vi "Process.vi"(8 "error in (no error)":errorcluster, 10 "Pound in":refnum<class "Pound.lvclass">, 11 "Qbus in":refnum<class "Qbus.lvclass">) -> (0 "error out":errorcluster)   [LabVIEW 2017, in "EmsaFPGABitfileManager.lvlib"]
uses:
  <vilib>/addons/InsightCM/Devices/Shared/Emsa/EmsaFPGABifileManager/EmsaFPGABitfileManager.lvlib
  <vilib>/addons/Qbus/Qbus.lvclass
  <vilib>/NI/Software Watchdog/Pound/Pound.lvclass
  <vilib>/addons/InsightCM/Devices/Shared/Emsa/EmsaFPGABifileManager/controls/config.ctl
  <vilib>/addons/TraceLogger/TraceLogger.lvlib
  <vilib>/NI/Software Watchdog/Watchdog/Watchdog.lvclass
  <vilib>/addons/InsightCM/Devices/Shared/Common/FpgaBitfileManager/FpgaBitfileManager.lvlib
  <vilib>/rvi/interface/nirviCloseFPGA/nirviCloseFPGA.xnode
  <vilib>/FPGAPlugInAG/Dynamic/niLvFpga_Close_Dynamic.vi
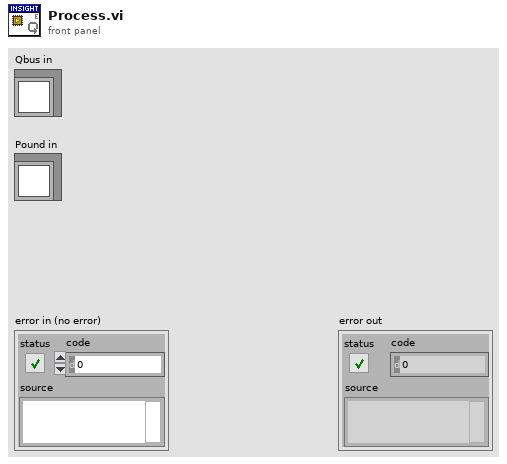
[diagram p1: front panel]
types:
  T1 = typedef "EmsaFPGABitfileManager.lvlib/config.ctl" = cluster{"FPGA VI Reference":refnum<k20>}
  T2 = typedef "cRIODetectHW.lvlib/SystemHW.ctl" = cluster{"controller":T3, "chassis":T3, "modules":T3[]}
  T3 = typedef "cRIODetectHW.lvlib/cRIO Product Info.ctl" = cluster{"vendorName":string, "productName":string, "serialNumber":string}
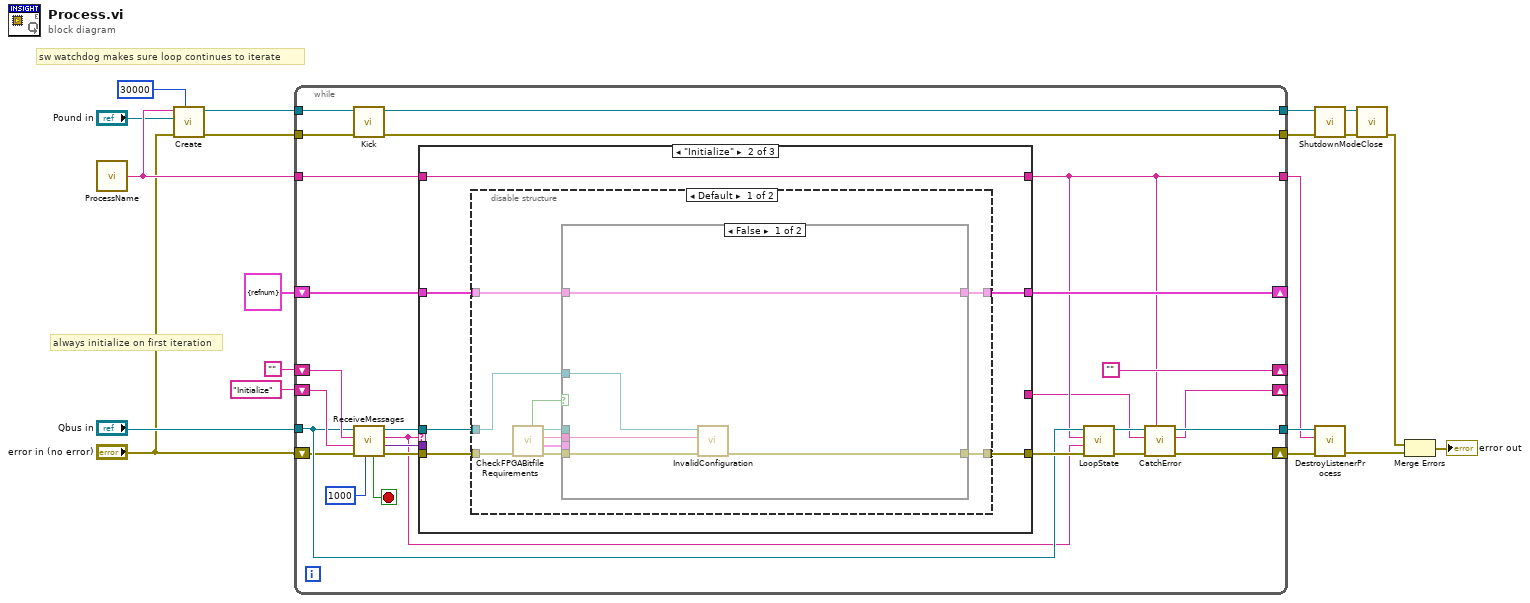
[diagram p0: block diagram]
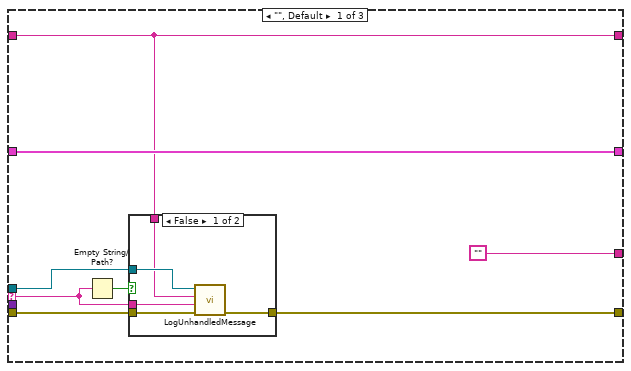
[diagram p2: hidden frame]
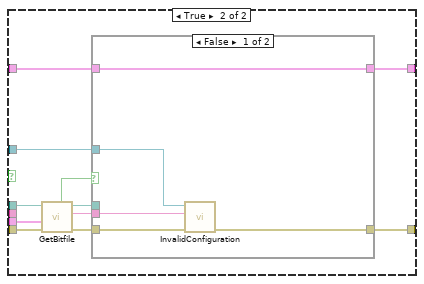
[diagram p4: hidden frame]
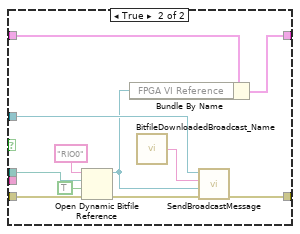
[diagram p5: hidden frame]
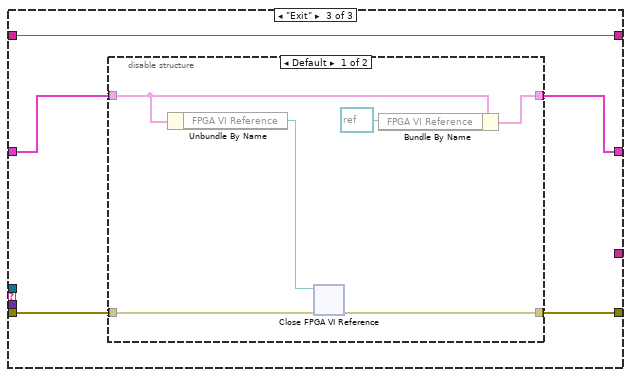
[diagram p7: hidden frame]
diagram:
  # "always initialize on first iteration"
  # "sw watchdog makes sure loop continues to iterate"
  n1 = call <vilib>:"ProcessName.vi"() -> ("process name"=w14:string)  [unwired: 5 in]
  n2 = call <vilib>:"Create.vi"("Execution Timeout (ms)"=u32 30000, "error in (no error)"="error in (no error)", "Pound"="Pound in", "Name"=w14) -> ("error out"=w7:errorcluster, "Watchdog"=w13:refnum<data-value>)  [unwired: 6 in]
  n3 = while {
    shift-right: [""] -> _
    shift-left: "" -> [w45]
    tunnel: "Qbus in" -> [w33]
    tunnel: w14 -> [w23]
    tunnel: [w36] -> w18
    tunnel: [w22] -> w17
    shift-right: [w35] -> _
    shift-left: "Initialize" -> [w40]
    shift-right: [w38] -> _
    shift-left: T1 {"FPGA VI Reference"=refnum} ("config") -> [w39]
    tunnel: w13 -> [w32]
    tunnel: [w31] -> w9
    tunnel: w7 -> [w30]
    tunnel: [w28] -> w6
    shift-right: [w37] -> w19
    shift-left: "error in (no error)" -> [w29]
    stop <- w46 stop-if-true
    n4 = call <vilib>:"Kick.vi"("error in (no error)"=w30, "Watchdog"=w32) -> ("error out"=w28:errorcluster, "Watchdog"=w31:refnum<data-value>)  [unwired: 8 in]
    n5 = call <vilib>:"ReceiveMessages.vi"("Timeout(1000)"=1000 ("milliseconds to wait"), "error in (no error)"=w29, "priority action"=w40, "default action"=w45, "Qbus in"=w33) -> ("error out"=w44:errorcluster, "message value"=w41:variant, "action"=w27:string, "Qbus out"=w42:refnum<class "Qbus.lvclass">, "exit"=w46:bool)  [unwired: 2 in]
    n6 = case shown="\"Initialize\"" w27 {
      selector: w27 -> [w51 _ _]
      tunnel: w44 -> [w53 w61 w114]
      tunnel: w42 -> [w49 w64 _]
      tunnel: [w52 w65 w113] -> w34
      tunnel: w41 -> [_ _ _]
      tunnel: w39 -> [w54 w63 w112]
      tunnel: [w54 w62 w111] -> w38
      tunnel: [w47 w66 w115] -> w22
      tunnel: w23 -> [w47 w66 w115]
      tunnel: ["" _ _] -> w21
      frame "", Default {
        n7 = Empty String/Path?(string/path=w51) -> (empty?=w50:bool)
        n8 = case shown="False" w50 {
          tunnel: [w58 w60] -> w52
          tunnel: w53 -> [w59 w60]
          tunnel: w51 -> [w56 _]
          tunnel: w49 -> [w57 _]
          tunnel: w47 -> [w55 _]
          frame False {
            n9 = call <vilib>:"LogUnhandledMessage.vi"("error in (no error)"=w59, "message"=w56, "process"=w55, "Qbus in"=w57) -> ("error out"=w58:errorcluster)  [unwired: 7 in]
          }
          frame True {
          }
        }
      }
      frame "Initialize" {
        n10 = disable-structure shown="Default" {
          disable-tunnel: [w76 w109] -> w65
          disable-tunnel: w64 -> [w75 _]
          disable-tunnel: w63 -> [w68 w110]
          disable-tunnel: [w67 w110] -> w62
          disable-tunnel: w61 -> [w74 w109]
          frame condition #0 {
            n11 = call <vilib>:"CheckFPGABitfileRequirements.vi"("error in (no error)"=w74) -> ("error out"=w73:errorcluster, "system info"=w69:T2, "description"=w72:string, "bitfile dir"=w70:path, "valid"=w71:bool)  [unwired: 6 in]
            n12 = case shown="False" w71 {
              tunnel: [w78 w92] -> w76
              tunnel: w75 -> [w79 w91]
              tunnel: w73 -> [w80 w90]
              tunnel: w72 -> [w81 _]
              tunnel: w70 -> [_ w88]
              tunnel: w69 -> [_ w87]
              tunnel: w68 -> [w77 w85]
              tunnel: [w77 w84] -> w67
              frame False {
                n13 = call <vilib>:"InvalidConfiguration.vi"("error in (no error)"=w80, "description"=w81, "Qbus in"=w79) -> ("error out"=w78:errorcluster)  [unwired: 7 in, 1 out]
              }
              frame True {
                n14 = call <vilib>:"GetBitfile.vi"("error in (no error)"=w90, "system info"=w87, "bitfile dir"=w88) -> ("error out"=w89:errorcluster, "error"=w86:string, "bitfile"=w82:path, "found"=w83:bool)  [unwired: 5 in]
                n15 = case shown="False" w83 {
                  tunnel: [w95 w107] -> w92
                  tunnel: w91 -> [w94 w106]
                  tunnel: w89 -> [w96 w102]
                  tunnel: w86 -> [w93 _]
                  tunnel: w85 -> [w97 w101]
                  tunnel: [w97 w100] -> w84
                  tunnel: w82 -> [_ w98]
                  frame False {
                    n16 = call <vilib>:"InvalidConfiguration.vi"("error in (no error)"=w96, "description"=w93, "Qbus in"=w94) -> ("error out"=w95:errorcluster)  [unwired: 7 in, 1 out]
                  }
                  frame True {
                    n17 = Open Dynamic Bitfile Reference(0:"RIO0" ("Device address"), 1:w98, 2:TRUE ("Run When Loaded"), 3:w102) -> (5:w99:refnum<k20>, 8:w105:errorcluster)  [unwired: 1 in]
                    n18 = Bundle By Name(cluster=w101, "FPGA VI Reference"=w99) -> (w100:T1)
                    n19 = call <vilib>:"BitfileDownloadedBroadcast_Name.vi"() -> ("message name"=w108:string)  [unwired: 5 in]
                    n20 = call <vilib>:"SendBroadcastMessage.vi"("error in (no error)"=w105, "message value"=w99, "message name"=w108, "Qbus in"=w106) -> ("error in (no error)"=w107:errorcluster)  [unwired: 6 in, 1 out]
                  }
                }
              }
            }
          }
          frame condition #1 (active) {
          }
        }
      }
      frame "Exit" {
        n21 = disable-structure shown="Default" {
          disable-tunnel: w114 -> [w121 w122]
          disable-tunnel: [w120 w122] -> w113
          disable-tunnel: w112 -> [w119 w123]
          disable-tunnel: [w118 w123] -> w111
          frame condition #0 {
            n22 = Unbundle By Name(w119) -> ("FPGA VI Reference"=w117:refnum<k20>)
            n23 = xnode "Close FPGA VI Reference"("FPGA VI Reference In"=w117, "error in"=w121) -> ("error out"=w120:errorcluster)
            n24 = Bundle By Name(cluster=w119, "FPGA VI Reference"=refnum<k20> refnum) -> (w118:T1)
          }
          frame condition #1 (active) {
          }
        }
      }
    }
    n25 = call <vilib>:"LoopState.vi"("error in (no error)"=w34, "loop action"=w27, "process name"=w22, "Qbus in"=w33) -> ("error out"=w25:errorcluster, "Qbus out"=w24:refnum<class "Qbus.lvclass">)  [unwired: 6 in]
    n26 = call <vilib>:"CatchError.vi"("source"=w22, "error in (no error)"=w25, "next action in"=w21, "Qbus in"=w24) -> ("error out"=w37:errorcluster, "next action out"=w35:string, "Qbus out"=w36:refnum<class "Qbus.lvclass">)  [unwired: 5 in]
  }
  n27 = call <vilib>:"ShutdownMode.vi"("error in (no error)"=w6, "Watchdog"=w9) -> ("error out"=w8:errorcluster, "Watchdog"=w10:refnum<data-value>)  [unwired: 8 in]
  n28 = call <vilib>:"DestroyListenerProcess.vi"("error in (no error)"=w19, "process name"=w17, "Qbus in"=w18) -> ("error in (no error)"=w5:errorcluster)  [unwired: 7 in, 1 out]
  n29 = call <vilib>:"Close.vi"("error in (no error)"=w8, "Watchdog"=w10) -> ("error out"=w4:errorcluster)  [unwired: 9 in]
  n30 = Merge Errors(w4, w5) -> (→"error out":errorcluster)
